vi "AgB29xx_LabVIEW_ListPulsedSweep.vi"() -> ()   [LabVIEW 2009]
panel:
  out "Items":string
  out "Simulate":bool
  out "SerialNumber":string
  out "Identifier":string
  out "Revision":string
  out "Vendor":string
  out "Description":string
  out "InstrumentModel":string
  out "InstrumentFirmwareRevision":string
  in  "OptionString":string="QueryInstrStatus=true, Simulate=true, DriverSetup= Model=, Trace=false"
  in  "Reset":bool=TRUE
  in  "IdQuery":bool=TRUE
  in  "ResourceName":string="GPIB0::23::INSTR"
  in  "APERTURE_TIME":dbl=0.0001
  in  "PULSE_WIDTH":dbl=0.001
  in  "PULSE_DELAY":dbl=0.0005
  out "iNumberOfChannels":i32=2
  out "data":dbl[](array[numeric])
  in  "AgB29xxLib.IAgB29xx2":refnum<k7>
  # "List Pulsed Sweep"
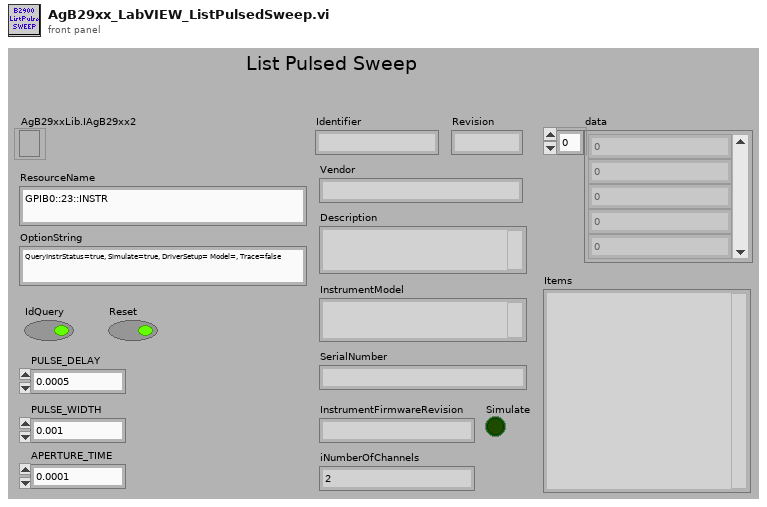
[diagram p1: front panel]
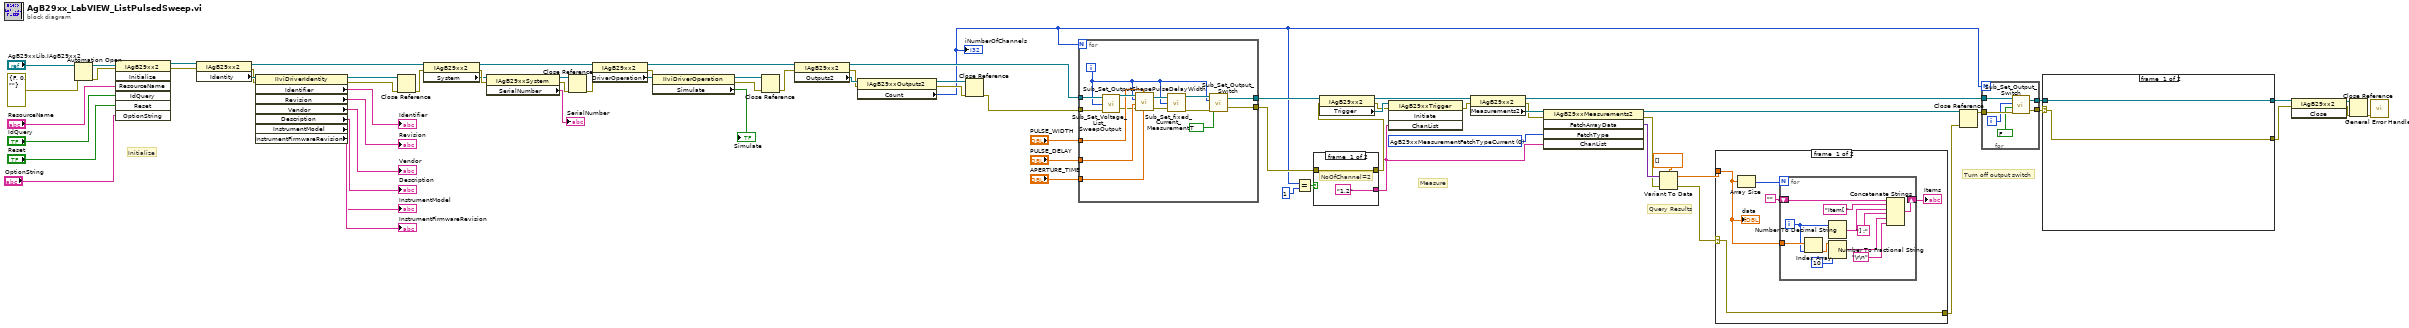
[diagram p0: block diagram]
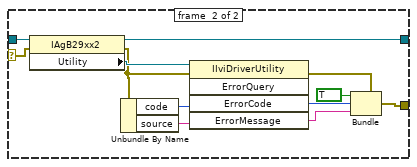
[diagram p2: hidden frame]
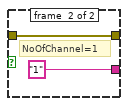
[diagram p4: hidden frame]
diagram:
  w24 = 0 items=["AgB29xxMeasurementFetchTypeCurrent", "AgB29xxMeasurementFetchTypeResistance", "AgB29xxMeasurementFetchTypeSource", "AgB29xxMeasurementFetchTypeStatus", "AgB29xxMeasurementFetchTypeTime", "AgB29xxMeasurementFetchTypeVoltage", "AgB29xxMeasurementFetchTypeAll"] ("FetchType")
  # "Turn off output switch"
  # "Query Results"
  # "Measure"
  # "Initialize"
  n1 = Automation Open(error in (no error)=errorcluster {"status"=FALSE, "code"=0, "source"=""}, Automation Refnum="AgB29xxLib.IAgB29xx2") -> (Automation Refnum=w73:refnum<k7>, error out=w74:errorcluster)  [unwired: 2 in]
  n2 = invoke class="IAgB29xx2" method="Initialize"(reference=w73, error in=w74, "ResourceName"="ResourceName", "IdQuery"="IdQuery", "Reset"="Reset", "OptionString"="OptionString") -> (reference out=w40:refnum<k7>, error out=w39:errorcluster)  [unwired: 1 in, 5 out]
  n3 = property class="IAgB29xx2"(reference=w40, error in=w39) -> (reference out=w60:refnum<k7>, error out=w63:errorcluster, "Identity"=w64:refnum<k7>)
  n4 = property class="IIviDriverIdentity"(reference=w64, error in=w63) -> (reference out=w59:refnum<k7>, error out=w58:errorcluster, "Identifier"=→"Identifier":string, "Revision"=→"Revision":string, "Vendor"=→"Vendor":string, "Description"=→"Description":string, "InstrumentModel"=→"InstrumentModel":string, "InstrumentFirmwareRevision"=→"InstrumentFirmwareRevision":string)
  n5 = Close Reference(reference=w59, error in (no error)=w58) -> (error out=w57:errorcluster)
  n6 = property class="IAgB29xx2"(reference=w60, error in=w57) -> (reference out=w54:refnum<k7>, error out=w62:errorcluster, "System"=w61:refnum<k7>)
  n7 = property class="IAgB29xxSystem"(reference=w61, error in=w62) -> (reference out=w52:refnum<k7>, error out=w53:errorcluster, "SerialNumber"=→"SerialNumber":string)
  n8 = Close Reference(reference=w52, error in (no error)=w53) -> (error out=w51:errorcluster)
  n9 = property class="IAgB29xx2"(reference=w54, error in=w51) -> (reference out=w34:refnum<k7>, error out=w55:errorcluster, "DriverOperation"=w56:refnum<k7>)
  n10 = property class="IIviDriverOperation"(reference=w56, error in=w55) -> (reference out=w50:refnum<k7>, error out=w49:errorcluster, "Simulate"=→"Simulate":bool)
  n11 = Close Reference(reference=w50, error in (no error)=w49) -> (error out=w33:errorcluster)
  n12 = property class="IAgB29xx2"(reference=w34, error in=w33) -> (reference out=w32:refnum<k7>, error out=w36:errorcluster, "Outputs2"=w38:refnum<k7>)
  n13 = property class="IAgB29xxOutputs2"(reference=w38, error in=w36) -> (reference out=w37:refnum<k7>, error out=w35:errorcluster, "Count"=w1:i32)
  "iNumberOfChannels" <- w1
  n14 = Close Reference(reference=w37, error in (no error)=w35) -> (error out=w31:errorcluster)
  n15 = for {
    N: w1 -> [_]
    tunnel: "PULSE_DELAY" -> [w89]
    tunnel: "PULSE_WIDTH" -> [w88]
    tunnel: "APERTURE_TIME" -> [w87]
    tunnel: w32 -> [w80]
    tunnel: w31 -> [w79]
    tunnel: [w78] -> w4
    tunnel: [w77] -> w3
    i -> [w76]
    n16 = call "Sub_Set_Voltage_List_SweepOutput.vi"("error in (no error)"=w79, "i"=w76, "AgB29xxLib.IAgB29xx2"=w80) -> ("error out"=w82:errorcluster, "AgB29xxLib.IAgB29xx2 2"=w90:refnum<k7>)
    n17 = call "Sub_Set_OutputShapePulseDelayWidth.vi"("APERTURE_TIME"=w87, "PULSE_WIDTH"=w88, "error in (no error)"=w82, "PULSE_DELAY"=w89, "i"=w76, "AgB29xxLib.IAgB29xx2"=w90) -> ("error out"=w85:errorcluster, "AgB29xxLib.IAgB29xx2 2"=w86:refnum<k7>)
    n18 = call "Sub_Set_fixed_Current_Measurement.vi"("error in"=w85, "i"=w76, "AgB29xxLib.IAgB29xx2"=w86) -> ("error out"=w83:errorcluster, "AgB29xxLib.IAgB29xx2 2"=w84:refnum<k7>)
    n19 = call "Sub_Set_Output_Switch.vi"("error in"=w83, "Enabled? (False)"=TRUE, "i"=w76, "AgB29xxLib.IAgB29xx2"=w84) -> ("error out"=w77:errorcluster, "AgB29xxLib.IAgB29xx2 2"=w78:refnum<k7>)
  }
  n20 = Equal?(x=w1, y=1 ("iStart")) -> (x = y?=w14:bool)
  n21 = case shown="False" w14 {
    tunnel: ["1,2" "1"] -> w12
    tunnel: w3 -> [w91 w93]
    tunnel: [w91 w93] -> w2
    frame #0 {
      # "NoOfChannel=2"
    }
    frame #1 {
      # "NoOfChannel=1"
    }
  }
  n22 = property class="IAgB29xx2"(reference=w4, error in=w2) -> (reference out=w26:refnum<k7>, error out=w21:errorcluster, "Trigger"=w28:refnum<k7>)
  n23 = invoke class="IAgB29xxTrigger" method="Initiate"(reference=w28, error in=w21, "ChanList"=w12) -> (error out=w25:errorcluster)  [unwired: 1 in, 3 out]
  n24 = property class="IAgB29xx2"(reference=w26, error in=w25) -> (reference out=w18:refnum<k7>, error out=w20:errorcluster, "Measurements2"=w27:refnum<k7>)
  n25 = invoke class="IAgB29xxMeasurements2" method="FetchArrayData"(reference=w27, error in=w20, "FetchType"=w24, "ChanList"=w12) -> (reference out=w19:refnum<k7>, error out=w15:errorcluster, "FetchArrayData"=w22:variant)  [unwired: 1 in, 2 out]
  n26 = Variant To Data(error in=w15, Variant=w22, type=dbl[] []) -> (error out=w10:errorcluster, data=w11:dbl[])
  n27 = case shown="No Error" w10 {
    selector: w10 -> [w97 w111]
    tunnel: w11 -> [w95 _]
    tunnel: [w97 w111] -> w9
    frame #0 {
      n28 = Array Size(array=w95) -> (size(s)=w96:i32)
      n29 = for {
        N: w96 -> [_]
        tunnel: w95 -> [w106]
        shift-right: [w103] -> w99
        shift-left: "" -> [w102]
        i -> [w101]
        n30 = Index Array(array=w106, index=w101) -> (element=w105:dbl)
        n31 = Number To Decimal String(number=w101) -> (decimal integer string=w109:string)  [unwired: 1 in]
        n32 = Number To Fractional String(number=w105, precision (6)=i16 10) -> (F-format string=w107:string)  [unwired: 2 in]
        n33 = Concatenate Strings(w102, "Item[ " ("string"), w109, "] :" ("string"), w107, "\r\n") -> (w103:string)
      }
      "Items" <- w99
      "data" <- w95
    }
    frame #1 {
    }
  }
  n34 = Close Reference(reference=w19, error in (no error)=w9) -> (error out=w17:errorcluster)
  n35 = for {
    N: w1 -> [_]
    tunnel: w18 -> [w117]
    tunnel: w17 -> [w116]
    tunnel: [w114] -> w8
    tunnel: [w113] -> w7
    i -> [w112]
    n36 = call "Sub_Set_Output_Switch.vi"("error in"=w116, "Enabled? (False)"=FALSE ("AutoRangeEnabled"), "i"=w112, "AgB29xxLib.IAgB29xx2"=w117) -> ("error out"=w114:errorcluster, "AgB29xxLib.IAgB29xx2 2"=w113:refnum<k7>)
  }
  n37 = case shown="Error" w8 {
    selector: w8 -> [w118 w130]
    tunnel: [w118 w120] -> w5
    tunnel: w7 -> [w119 w131]
    tunnel: [w119 w128] -> w6
    frame #0 {
    }
    frame #1 {
      n38 = property class="IAgB29xx2"(reference=w131, error in=w130) -> (reference out=w128:refnum<k7>, error out=w125:errorcluster, "Utility"=w129:refnum<k7>)
      n39 = Unbundle By Name(w125) -> ("code"=w127:i32, "source"=w126:string)
      n40 = invoke class="IIviDriverUtility" method="ErrorQuery"(reference=w129, error in=w125, "ErrorCode"=w127, "ErrorMessage"=w126) -> (error out=w121:errorcluster, "ErrorCode"=w124:i32, "ErrorMessage"=w123:string)  [unwired: 1 in, 2 out]
      n41 = Bundle(cluster=w121, "status"=TRUE, "code"=w124, "source"=w123) -> (w120:errorcluster)
    }
  }
  n42 = invoke class="IAgB29xx2" method="Close"(reference=w6, error in=w5) -> (reference out=w30:refnum<k7>, error out=w29:errorcluster)  [unwired: 1 in, 1 out]
  n43 = Close Reference(reference=w30, error in (no error)=w29) -> (error out=w16:errorcluster)
  n44 = call <vilib>:"General Error Handler.vi"("error in (no error)"=w16) -> ()  [unwired: 10 in, 5 out]
